vi "Coords_to_Index.vi"(8 "error in (no error)":errorcluster, 9 "coords":cluster{"Horizontal":i32, "Vertical":i32}, 11 "Array ref":refnum<vi>) -> (0 "error out":errorcluster, 1 "col index":i16, 2 "H In Range?":bool, 3 "row index":i16, 5 "V In Range?":bool)   [LabVIEW 2020]
doc: "Given a reference to a 1-D or 2-D array, and screen coordinates,\nreturn the index of the element at that location.\nTwo values are returned: col index is valid for horizontal arrays, and row index is valid for vertical arrays, both are valid for 2-D arrays"
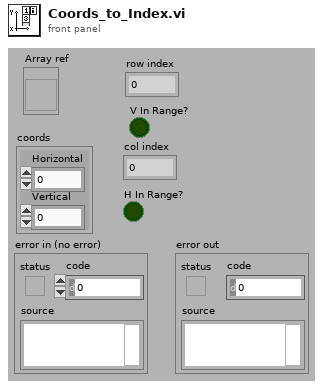
[diagram p1: front panel]
types:
  T1 = typedef "LVRectTypeDef.ctl" = cluster{"Left":i16, "Top":i16, "Right":i16, "Bottom":i16}
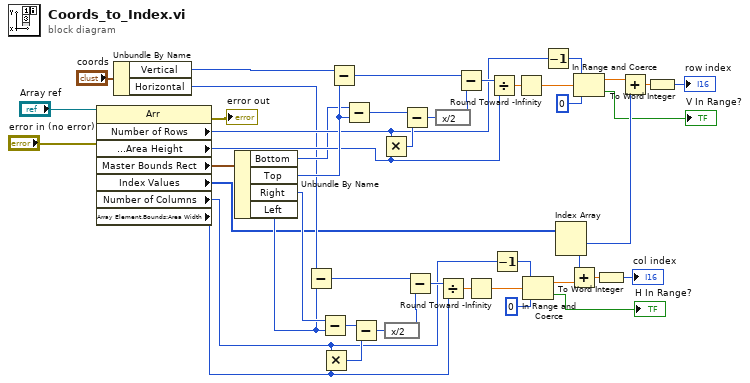
[diagram p0: block diagram]
diagram:
  n1 = property on="Property Node" class="Arr"(reference="Array ref", error in="error in (no error)") -> (error out=→"error out":errorcluster, "Number of Rows"=w8:u32, "Array Element.Bounds:Area Height"=w15:u32, "Master Bounds Rect"=w7:T1, "Index Values"=w3:u32[], "Number of Columns"=w11:u32, "Array Element.Bounds:Area Width"=w10:u32)  [unwired: 1 out]
  n2 = Unbundle By Name("coords") -> ("Vertical"=w41:i32, "Horizontal"=w4:i32)
  n3 = Unbundle By Name(w7) -> ("Bottom"=w6:i16, "Top"=w17:i16, "Right"=w12:i16, "Left"=w5:i16)
  n4 = Subtract(x=w4, y=w5) -> (x-y=w27:i32)
  n5 = Subtract(x=w12, y=w5) -> (x-y=w14:i16)
  n6 = Multiply(x=w11, y=w10) -> (x*y=w30:u32)
  n7 = Subtract(x=w41, y=w17) -> (x-y=w22:i32)
  n8 = Subtract(x=w6, y=w17) -> (x-y=w16:i16)
  n9 = Subtract(x=w14, y=w30) -> (x-y=w29:u32)
  n10 = Multiply(x=w8, y=w15) -> (x*y=w24:u32)
  n11 = expression code="x/2"(w29) -> (w28:u32)
  n12 = Subtract(x=w16, y=w24) -> (x-y=w25:u32)
  n13 = Subtract(x=w27, y=w28) -> (x-y=w26:u32)
  n14 = expression code="x/2"(w25) -> (w23:u32)
  n15 = Divide(x=w26, y=w10) -> (x/y=w33:dbl)
  n16 = Subtract(x=w22, y=w23) -> (x-y=w21:u32)
  n17 = Round Toward -Infinity(1:w33) -> (0:w19:dbl)
  n18 = Divide(x=w21, y=w15) -> (x/y=w34:dbl)
  n19 = Decrement(x=w11) -> (x-1=w38:u32)
  n20 = Round Toward -Infinity(1:w34) -> (0:w20:dbl)
  n21 = In Range and Coerce(upper limit=w38, x=w19, lower limit=u32 0) -> (coerced(x)=w2:dbl, In Range?=→"H In Range?":bool)
  n22 = Decrement(x=w8) -> (x-1=w43:u32)
  n23 = Index Array(array=w3) -> (element #1=w45:u32, element #2=w1:u32)  [unwired: 2 in]
  n24 = Add(x=w1, y=w2) -> (x+y=w39:dbl)
  n25 = In Range and Coerce(upper limit=w43, x=w20, lower limit=u32 0) -> (coerced(x)=w46:dbl, In Range?=→"V In Range?":bool)
  n26 = To Word Integer(number=w39) -> (16bit integer=→"col index":i16)
  n27 = Add(x=w46, y=w45) -> (x+y=w44:dbl)
  n28 = To Word Integer(number=w44) -> (16bit integer=→"row index":i16)
